vi "CreateSweep.vi"(9 "Max":dbl format="%#_13g", 10 "Step":dbl format="%#_13g", 11 "Init Value":dbl format="%#_13g") -> (2 "Array":dbl[](array[numeric]))   [LabVIEW 2014]
panel:
  out "appended array":dbl[][](array[numeric])
  out "element":dbl
  out "x/y":dbl
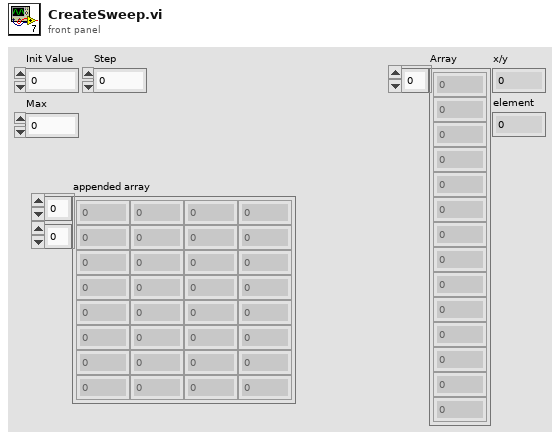
[diagram p1: front panel]
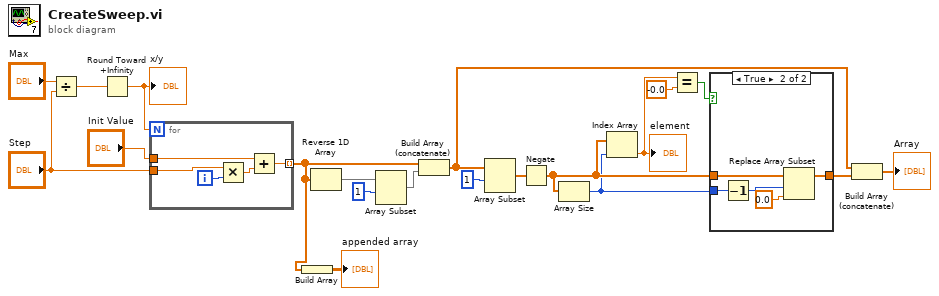
[diagram p0: block diagram]
diagram:
  n1 = Divide(x="Max", y="Step") -> (x/y=w17:dbl)
  n2 = Round Toward +Infinity(x=w17) -> (ceil(x): smallest int >= x=w6:dbl)
  "x/y" <- w6
  n3 = for {
    N: w6 -> [_]
    tunnel: "Step" -> [w24]
    tunnel: "Init Value" -> [w22]
    tunnel: [w21] -> w2 mode=indexing
    i -> [w25]
    n4 = Multiply(x=w24, y=w25) -> (x*y=w23:dbl)
    n5 = Add(x=w22, y=w23) -> (x+y=w21:dbl)
  }
  n6 = Build Array(w2) -> (→"appended array":dbl[][])
  n7 = Reverse 1D Array(array=w2) -> (reversed array=w15:dbl[])
  n8 = Array Subset(array=w15, index=1) -> (w14:dbl[])  [unwired: 1 in]
  n9 = Build Array (concatenate)(w2, w14) -> (w4:dbl[])
  n10 = Array Subset(array=w4, index=1) -> (w3:dbl[])  [unwired: 1 in]
  n11 = Negate(x=w3) -> (-x=w9:dbl[])
  n12 = Array Size(array=w9) -> (size(s)=w8:i32)
  n13 = Index Array(array=w9, index=w8) -> (element=w12:dbl)
  "element" <- w12
  n14 = Equal?(x=w12, y=-0.0) -> (x = y?=w10:bool)
  n15 = case shown="True" w10 {
    tunnel: w9 -> [w26 w31]
    tunnel: w8 -> [_ w30]
    tunnel: [w26 w28] -> w7
    frame False {
    }
    frame True {
      n16 = Decrement(x=w30) -> (x-1=w27:i32)
      n17 = Replace Array Subset(array=w31, new element=0.0 ("new element/subarray"), index=w27) -> (w28:dbl[])
    }
  }
  n18 = Build Array (concatenate)(w4, w7) -> (→"Array":dbl[])
